vi "controlRtOutMode.vi"(7 "set":bool, 8 "error in":errorcluster, 9 "RtOutMode":enum16{"Off", "AquadB", "Trigger"}(ring), 10 "axis":i32, 11 "connection ID":refnum<k5>) -> (0 "error out":errorcluster, 1 "RtOutMode":enum16{"Off", "AquadB", "Trigger"}(ring), 2 "axis_out":i32, 3 "connection ID":refnum<k5>)   [LabVIEW 2016]
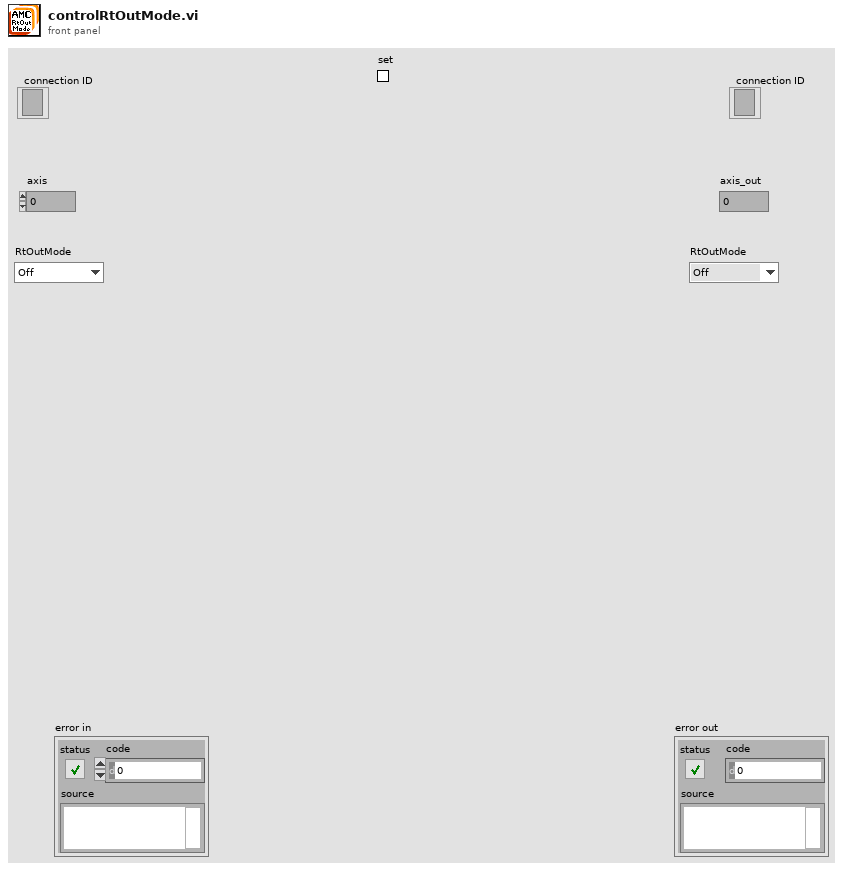
[diagram p1: front panel]
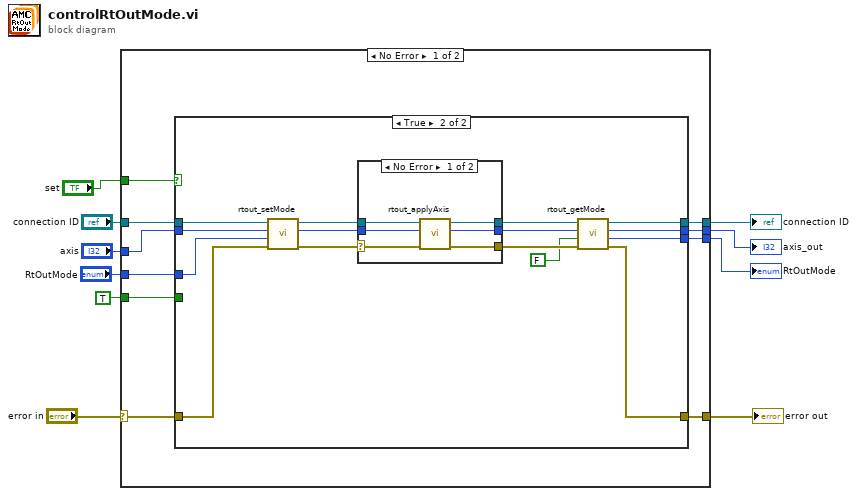
[diagram p0: block diagram]
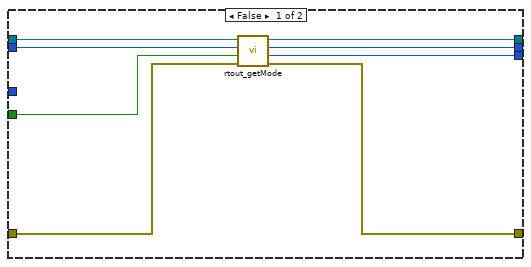
[diagram p2: hidden frame]
diagram:
  n1 = case shown="No Error" "error in" {
    selector: "error in" -> [w13 w56]
    tunnel: [w14 w56] -> w10
    tunnel: [w18 w55] -> w9
    tunnel: "connection ID" -> [w19 w55]
    tunnel: "axis" -> [w16 w54]
    tunnel: TRUE ("tempvalue") -> [w17 _]
    tunnel: [w12 w53] -> w4
    tunnel: "set" -> [w20 _]
    tunnel: [w15 w54] -> w2
    tunnel: "RtOutMode" -> [w11 w53]
    frame No Error {
      n2 = case shown="True" w20 {
        tunnel: w19 -> [w28 w43]
        tunnel: [w27 w35] -> w18
        tunnel: w17 -> [w26 _]
        tunnel: w16 -> [w25 w41]
        tunnel: [w24 w31] -> w15
        tunnel: [w23 w34] -> w14
        tunnel: w13 -> [w22 w42]
        tunnel: [w21 w30] -> w12
        tunnel: w11 -> [_ w40]
        frame False {
          n3 = call "rtout_getMode.vi"("error in"=w22, "tempvalue"=w26, "axis"=w25, "connection ID"=w28) -> ("error out"=w23:errorcluster, "mode"=w21:i32, "axis_out"=w24:i32, "connection ID"=w27:refnum<k5>)  [unwired: 4 in]
        }
        frame True {
          n4 = call "rtout_setMode.vi"("error in"=w42, "mode"=w40, "axis"=w41, "connection ID"=w43) -> ("error out"=w37:errorcluster, "axis_out"=w38:i32, "connection ID"=w39:refnum<k5>)  [unwired: 5 in]
          n5 = case shown="No Error" w37 {
            selector: w37 -> [w45 w50]
            tunnel: w39 -> [w49 w52]
            tunnel: w38 -> [w48 w51]
            tunnel: [w47 w52] -> w36
            tunnel: [w46 w51] -> w33
            tunnel: [w44 w50] -> w32
            frame No Error {
              n6 = call "rtout_applyAxis.vi"("error in"=w45, "axis"=w48, "connection ID"=w49) -> ("error out"=w44:errorcluster, "axis_out"=w46:i32, "connection ID"=w47:refnum<k5>)  [unwired: 6 in]
            }
            frame Error {
            }
          }
          n7 = call "rtout_getMode.vi"("error in"=w32, "tempvalue"=FALSE, "axis"=w33, "connection ID"=w36) -> ("error out"=w34:errorcluster, "mode"=w30:i32, "axis_out"=w31:i32, "connection ID"=w35:refnum<k5>)  [unwired: 4 in]
        }
      }
    }
    frame Error {
    }
  }
  "error out" <- w10
  "connection ID" <- w9
  "axis_out" <- w2
  "RtOutMode" <- w4
